vi "实时小时数据单参数上传.vi"() -> (4 "数据发送起始时间":timestamp format="%<%.3X\n%Y/%m/%d>T", 15 "error out":errorcluster)   [LabVIEW 2016, in "数据传输系统-04.lvlib"]
uses:
  <vilib>/Utility/config.llb/Read Key (String).vi
  <vilib>/Utility/config.llb/Write Key (String).vi
  <vilib>/Utility/config.llb/NI_LVConfig.lvlib
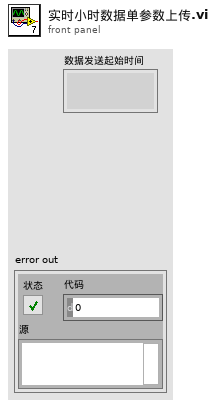
[diagram p1: front panel]
types:
  T1 = cluster{"CODMn":string, "CODCr":string, "DO":string, "铜":string, "PH":string, "氨氮":string, "比电导率":string, "水温":string, "COD":string, "浊度":string, "总氮":string, "总磷":string, "叶绿素a":string, "藻密度":string, "水位":string, "流速":string, "瞬时流量":string, "累积流量":string, "亚硝酸盐":string, "硫化物":string, "ORP":string, "铅":string, "镉":string, "锌":string, "镍":string, "锰":string, "汞":string, "气温":string, "气压":string, "风速":string, "风向":string, "盐度":string, "磷酸盐":string, "硝氮":string, "氟化物":string}
  T2 = cluster{"setini":string, "sysini":string, "hechaini":string, "actualwrite":string, "actualread":string, "datasent":string, "反控命令信息队列":string, "反控与仪器交互":string}
  T3 = typedef "NI_LVConfig.lvlib/Config Data RefNum.ctl" = refnum<k1>
  T4 = cluster{"time1":string, "time2":string, "time3":string, "time4":string, "time5":string, "time6":string, "time7":string, "time8":string, "time9":string, "time10":string, "time11":string, "time12":string, "time13":string, "time14":string, "time15":string, "time16":string, "time17":string, "time18":string, "time19":string, "time20":string, "time21":string, "time22":string, "time23":string, "time24":string, "time25":string, "time26":string, "time27":string, "time28":string, "time29":string, "time30":string, "time31":string, "time32":string, "time33":string, "time34":string, "time35":string}
  T5 = cluster{"水样数据索引[0]":string, "水样数据索引[1]":string, "水样数据索引[2]":string, "水样数据索引[3]":string, "水样数据索引[4]":string, "水样数据索引[5]":string, "水样数据索引[6]":string, "水样数据索引[7]":string, "水样数据索引[8]":string, "水样数据索引[9]":string, "水样数据索引[10]":string, "水样数据索引[11]":string, "水样数据索引[12]":string, "水样数据索引[13]":string, "水样数据索引[14]":string, "水样数据索引[15]":string, "水样数据索引[16]":string, "水样数据索引[17]":string, "水样数据索引[18]":string, "水样数据索引[19]":string, "水样数据索引[20]":string, "水样数据索引[21]":string, "水样数据索引[22]":string, "水样数据索引[23]":string, "水样数据索引[24]":string, "水样数据索引[25]":string, "水样数据索引[26]":string, "水样数据索引[27]":string, "水样数据索引[28]":string, "水样数据索引[29]":string, "水样数据索引[30]":string, "水样数据索引[31]":string, "水样数据索引[32]":string, "水样数据索引[33]":string, "水样数据索引[34]":string}
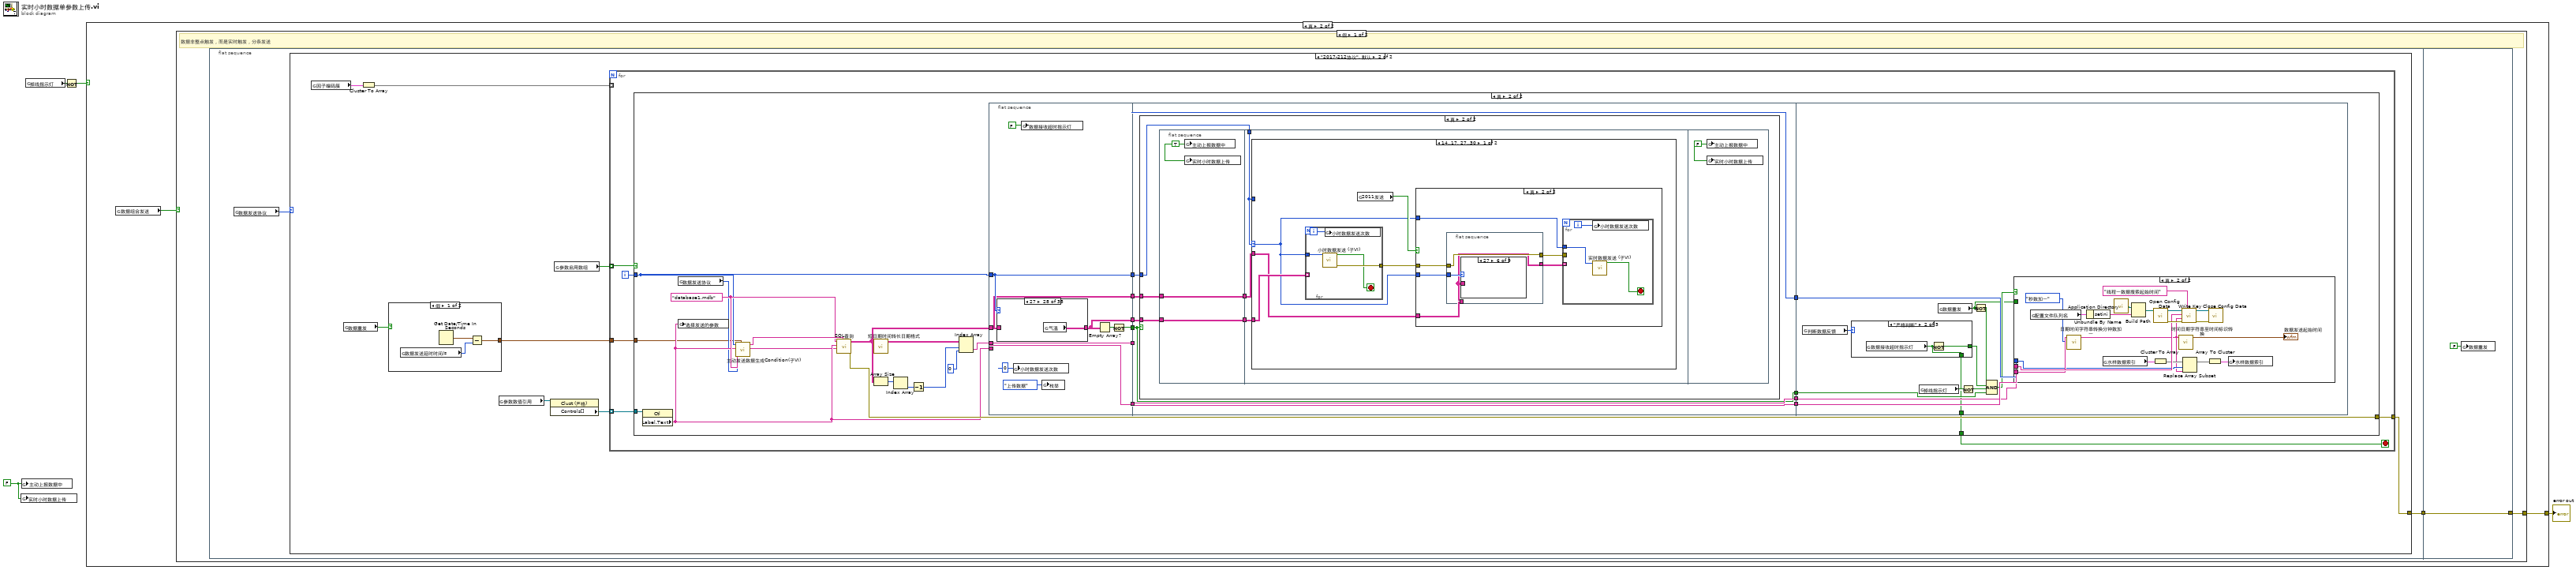
[diagram p0: block diagram]
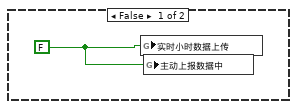
[diagram p2: hidden frame]
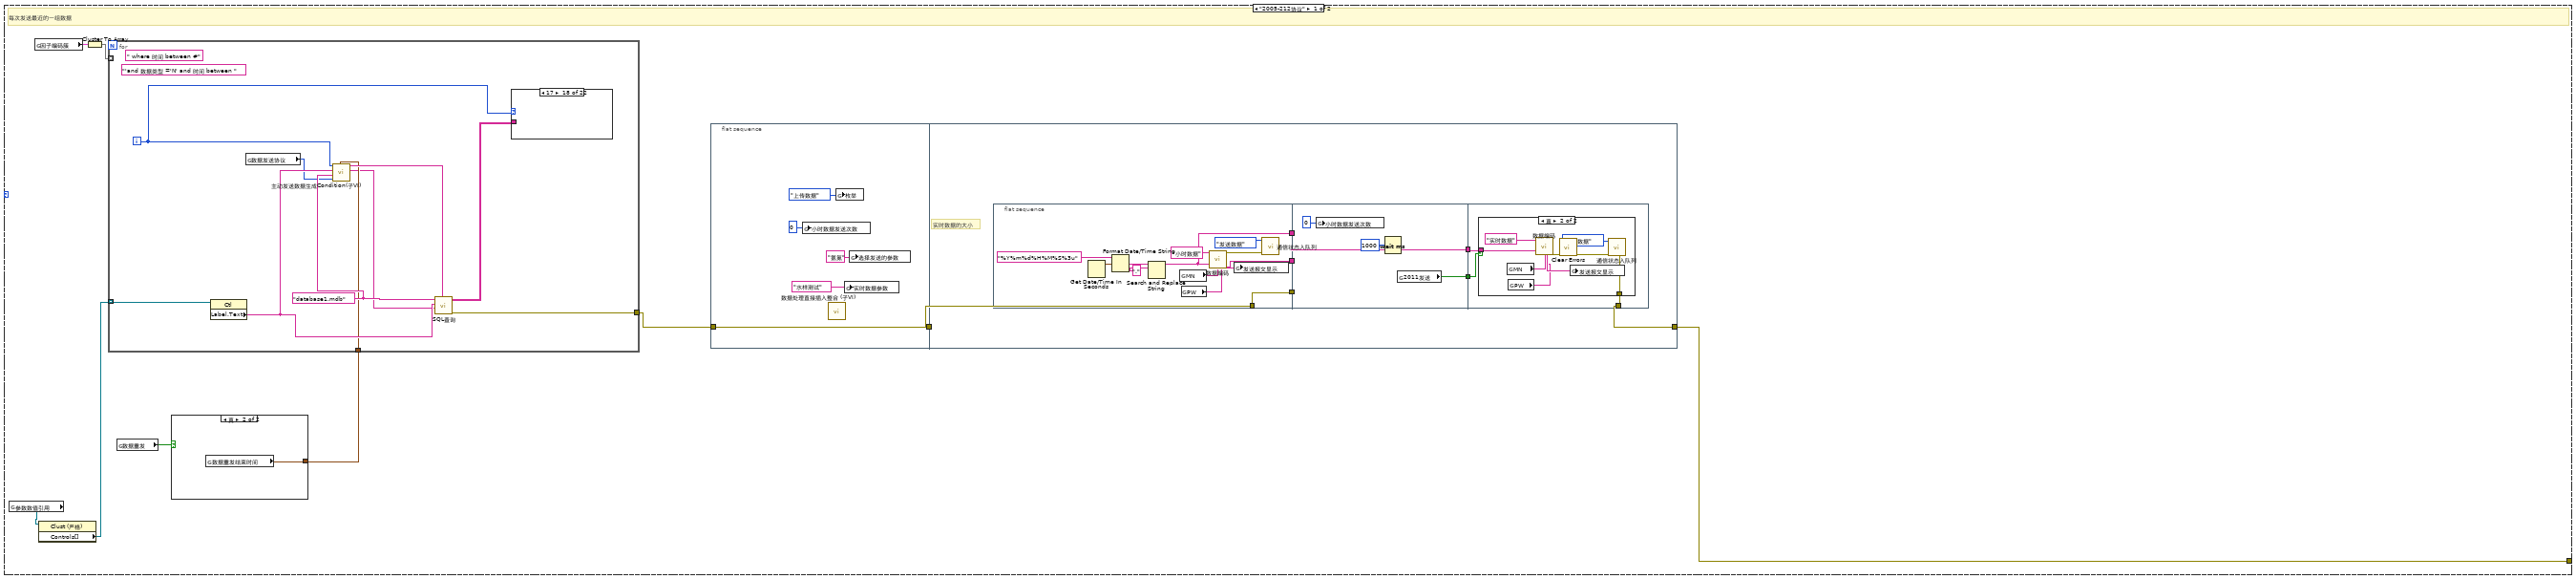
[diagram p3: hidden frame]
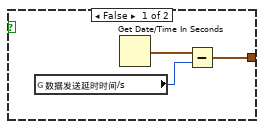
[diagram p4: hidden frame]
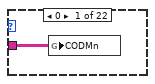
[diagram p6: hidden frame]
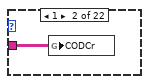
[diagram p7: hidden frame]
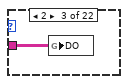
[diagram p8: hidden frame]
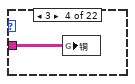
[diagram p9: hidden frame]
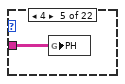
[diagram p10: hidden frame]
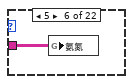
[diagram p11: hidden frame]
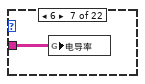
[diagram p12: hidden frame]
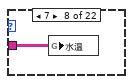
[diagram p13: hidden frame]
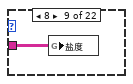
[diagram p14: hidden frame]
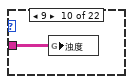
[diagram p15: hidden frame]
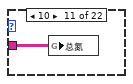
[diagram p16: hidden frame]
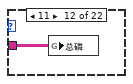
[diagram p17: hidden frame]
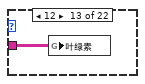
[diagram p18: hidden frame]
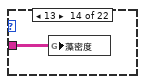
[diagram p19: hidden frame]
diagram:
  w1 = FALSE ("小时数据上传")
  n1 = global write "全局1.vi" "实时小时数据上传"(w1) -> ()
  n2 = global write "全局 数据发送重叠.vi" "主动上报数据中"(w1) -> ()
  n3 = global read "全局 数据发送重叠.vi" "掉线指示灯"() -> (w4:bool)
  n4 = Not(x=w4) -> (.not. x?=w3:bool)
  n5 = case shown="真" w3 {
    tunnel: [_ w7] -> w2
    frame False {
      w5 = FALSE ("小时数据上传")
      n6 = global write "全局1.vi" "实时小时数据上传"(w5) -> ()
      n7 = global write "全局 数据发送重叠.vi" "主动上报数据中"(w5) -> ()
    }
    frame True {
      n8 = global read "断电保存全局.vi" "数据组合发送"() -> (w6:bool)
      n9 = case shown="假" w6 {
        tunnel: [w8 _] -> w7
        frame False {
          # "数据非整点触发，而是实时触发，分条发送"
          n10 = flat-sequence {
            tunnel: [w11] -> w9
            tunnel: [w341] -> w8
            tunnel: w9 -> [w341]
            frame #0 {
              n11 = global read "断电保存全局.vi" "数据发送协议"() -> (w10:enum16{"2005-212协议", "2017-212协议"})
              n12 = case shown="\"2017-212协议\", 默认" w10 {
                tunnel: [w16 w98] -> w11
                frame "2005-212协议" {
                  # "每次发送最近的一组数据"
                  n13 = global read "断电保存全局.vi" "参数数值引用"() -> (w14:refnum<vi>)
                  n14 = global read "断电保存全局.vi" "因子编码簇"() -> (w15:T1)
                  n15 = property class="Clust (严格)"(reference=w14) -> ("Controls[]"=w17:refnum<vi>[])  [unwired: 1 in, 2 out]
                  n16 = Cluster To Array(cluster=w15) -> (array=w20:string[])
                  n17 = global read "断电保存全局.vi" "数据重发"() -> (w13:bool)
                  n18 = case shown="真" w13 {
                    tunnel: [w21 w24] -> w12
                    frame False {
                      n19 = global read "断电保存全局.vi" "数据发送延时时间/s"() -> (w22:i32)
                      n20 = Get Date/Time In Seconds() -> (seconds since 1Jan1904=w23:timestamp)
                      n21 = Subtract(x=w23, y=w22) -> (x-y=w21:timestamp)
                    }
                    frame True {
                      n22 = global read "断电保存全局.vi" "数据重发结束时间"() -> (w24:timestamp)
                    }
                  }
                  n23 = for {
                    tunnel: w20 -> [_] mode=indexing
                    tunnel: [w74] -> w19
                    tunnel: w17 -> [w69] mode=indexing
                    tunnel: w12 -> [w66]
                    i -> [w67]
                    (unwired) " where 时间 between #"
                    w72 = "database1.mdb" ("database")
                    (unwired) "'and 数据类型 ='N' and 时间 between "
                    n24 = property class="Ctl"(reference=w69) -> ("Label.Text"=w73:string)  [unwired: 1 in, 2 out]
                    n25 = global read "断电保存全局.vi" "数据发送协议"() -> (w70:enum16{"2005-212协议", "2017-212协议"})
                    n26 = call "主动发送数据生成Condition(子VI).vi"("结束时间"=w66, "数据发送协议"=w70, "database"=w72, "Label.Text"=w73, "数值"=w67) -> ("columns"=w65:string[], "CONDITION"=w71:string)  [unwired: 5 in]
                    n27 = call "SQL查询.vi"("condition"=w71, "columns"=w65, "table输入"=w73, "database"=w72) -> ("error out"=w74:errorcluster, "data"=w68:string[][])  [unwired: 5 in, 1 out]
                    n28 = case shown="17" w67 {
                      tunnel: w68 -> [w75 w76 w77 w78 w79 w80 w81 w82 w83 w84 w85 w86 w87 w88 _ _ _ _ w89 w90 w91 _]
                      frame 0 {
                        n29 = global write "全局 所有参数.vi" "CODMn"(w75) -> ()
                      }
                      frame 1 {
                        n30 = global write "全局 所有参数.vi" "CODCr"(w76) -> ()
                      }
                      frame 2 {
                        n31 = global write "全局 所有参数.vi" "DO"(w77) -> ()
                      }
                      frame 3 {
                        n32 = global write "全局 所有参数.vi" "铜"(w78) -> ()
                      }
                      frame 4 {
                        n33 = global write "全局 所有参数.vi" "PH"(w79) -> ()
                      }
                      frame 5 {
                        n34 = global write "全局 所有参数.vi" "氨氮"(w80) -> ()
                      }
                      frame 6 {
                        n35 = global write "全局 所有参数.vi" "电导率"(w81) -> ()
                      }
                      frame 7 {
                        n36 = global write "全局 所有参数.vi" "水温"(w82) -> ()
                      }
                      frame 8 {
                        n37 = global write "全局 所有参数.vi" "盐度"(w83) -> ()
                      }
                      frame 9 {
                        n38 = global write "全局 所有参数.vi" "浊度"(w84) -> ()
                      }
                      frame 10 {
                        n39 = global write "全局 所有参数.vi" "总氮"(w85) -> ()
                      }
                      frame 11 {
                        n40 = global write "全局 所有参数.vi" "总磷"(w86) -> ()
                      }
                      frame 12 {
                        n41 = global write "全局 所有参数.vi" "叶绿素"(w87) -> ()
                      }
                      frame 13 {
                        n42 = global write "全局 所有参数.vi" "藻密度"(w88) -> ()
                      }
                      frame 14 {
                      }
                      frame 15 {
                      }
                      frame 16 {
                      }
                      frame 17 {
                      }
                      frame 18 {
                        n43 = global write "全局 所有参数.vi" "亚硝酸盐"(w89) -> ()
                      }
                      frame 19 {
                        n44 = global write "全局 所有参数.vi" "硫化物"(w90) -> ()
                      }
                      frame 20 {
                        n45 = global write "全局 所有参数.vi" "ORP"(w91) -> ()
                      }
                      frame 21, Default {
                      }
                    }
                  }
                  n46 = flat-sequence {
                    tunnel: w19 -> [w25]
                    tunnel: [w25] -> w18
                    tunnel: w18 -> [w34]
                    tunnel: [w33] -> w16
                    frame #0 {
                      n47 = global write "全局 小时数据发送次数.vi" "小时数据发送次数"(0 ("小时数据发送次数")) -> ()
                      n48 = call "数据处理直接插入整合 (子VI).vi"() -> ()  [unwired: 12 in]
                      n49 = global write "全局1.vi" "枚举"(enum16{"返回请求应答", "上传数据", "返回执行结果"}."上传数据" ("枚举")) -> ()
                      n50 = global write "全局 实时数据参数.vi" "实时数据参数"("水样测试" ("实时数据参数")) -> ()
                      n51 = global write "全局 水样时间.vi" "选择发送的参数"("氨氮" ("选择发送的参数")) -> ()
                    }
                    frame #1 {
                      # "实时数据的大小"
                      n52 = flat-sequence {
                        tunnel: [w43] -> w36
                        tunnel: [w38] -> w35
                        tunnel: w34 -> [w38]
                        tunnel: [w37] -> w32
                        tunnel: w36 -> [_]
                        tunnel: w35 -> [_]
                        tunnel: w32 -> [w50]
                        tunnel: [w50] -> w31
                        tunnel: [w49] -> w30
                        tunnel: [w55] -> w33
                        tunnel: w31 -> [w54]
                        tunnel: w30 -> [w53]
                        frame #0 {
                          n53 = Get Date/Time In Seconds() -> (seconds since 1Jan1904=w46:timestamp)
                          n54 = Format Date/Time String(time format string (%c)="%Y%m%d%H%M%S%3u" ("时间格式字符串(%c)"), seconds (now)=w46) -> (date/time string=w47:string)  [unwired: 1 in]
                          n55 = Search and Replace String(input string=w47, search string="." ("搜索字符串")) -> (result string=w37:string)  [unwired: 6 in, 3 out]
                          n56 = global read "断电保存全局.vi" "MN"() -> (w41:string)
                          n57 = global read "断电保存全局.vi" "PW"() -> (w40:string)
                          n58 = call "数据编码.vi"("table输入"="小时数据" ("新元素/子数组"), "QN"=w37, "MN"=w41, "PW"=w40) -> ("错误常量"=w39:errorcluster, "通讯包字符串"=w43:string)  [unwired: 10 in]
                          n59 = global write "全局1.vi" "发送报文显示"(w43) -> ()
                          n60 = call "通信状态入队列.vi"("错误输入（无错误）"=w39, "枚举"=enum16{"打开连接", "发送数据", "读取数据", "数据处理", "关闭连接"}."发送数据") -> ()  [unwired: 9 in, 1 out]
                        }
                        frame #1 {
                          n61 = global write "全局 小时数据发送次数.vi" "小时数据发送次数"(0 ("小时数据发送次数")) -> ()
                          n62 = Wait (ms)(milliseconds to wait=u32 1000 ("等待时间（毫秒）")) -> ()  [unwired: 1 out]
                          n63 = global read "断电保存全局.vi" "2011发送"() -> (w49:bool)
                        }
                        frame #2 {
                          n64 = case shown="真" w53 {
                            tunnel: [_ w58] -> w55
                            tunnel: w54 -> [_ w57]
                            frame False {
                            }
                            frame True {
                              n65 = global read "断电保存全局.vi" "MN"() -> (w60:string)
                              n66 = global read "断电保存全局.vi" "PW"() -> (w61:string)
                              n67 = call "数据编码.vi"("table输入"="实时数据" ("新元素/子数组"), "QN"=w57, "MN"=w60, "PW"=w61) -> ("错误常量"=w59:errorcluster, "通讯包字符串"=w63:string)  [unwired: 10 in]
                              n68 = call <vilib>:"Clear Errors.vi"("error in (no error)"=w59) -> ("error out"=w56:errorcluster)  [unwired: 5 in, 1 out]
                              n69 = global write "全局1.vi" "发送报文显示"(w63) -> ()
                              n70 = call "通信状态入队列.vi"("错误输入（无错误）"=w56, "枚举"=enum16{"打开连接", "发送数据", "读取数据", "数据处理", "关闭连接"}."发送数据") -> ("错误输出"=w58:errorcluster)  [unwired: 9 in]
                            }
                          }
                        }
                      }
                    }
                  }
                }
                frame "2017-212协议", Default {
                  n71 = global read "断电保存全局.vi" "因子编码簇"() -> (w96:T1)
                  n72 = global read "断电保存全局.vi" "数据重发"() -> (w93:bool)
                  n73 = Cluster To Array(cluster=w96) -> (array=w99:string[])
                  n74 = case shown="假" w93 {
                    tunnel: [w100 w103] -> w92
                    frame False {
                      n75 = global read "断电保存全局.vi" "数据发送延时时间/s"() -> (w101:i32)
                      n76 = Get Date/Time In Seconds() -> (seconds since 1Jan1904=w102:timestamp)
                      n77 = Subtract(x=w102, y=w101) -> (x-y=w100:timestamp)
                    }
                    frame True {
                      n78 = global read "断电保存全局.vi" "数据重发结束时间"() -> (w103:timestamp)
                    }
                  }
                  n79 = global read "断电保存全局.vi" "参数数值引用"() -> (w95:refnum<vi>)
                  n80 = property class="Clust (严格)"(reference=w95) -> ("Controls[]"=w97:refnum<vi>[])  [unwired: 1 in, 2 out]
                  n81 = global read "断电保存全局.vi" "参数启用数组"() -> (w94:bool[])
                  n82 = for {
                    tunnel: w99 -> [_] mode=indexing
                    tunnel: [w109] -> w98
                    tunnel: w97 -> [w107] mode=indexing
                    tunnel: w94 -> [w106] mode=indexing
                    tunnel: w92 -> [w105]
                    i -> [w108]
                    stop <- w104 stop-if-true
                    n83 = case shown="真" w106 {
                      tunnel: [_ w125] -> w109
                      tunnel: w108 -> [_ w116]
                      tunnel: w107 -> [_ w115]
                      tunnel: w105 -> [_ w112]
                      tunnel: [_ w110] -> w104
                      frame False {
                      }
                      frame True {
                        w124 = "database1.mdb" ("database")
                        n84 = property class="Ctl"(reference=w115) -> ("Label.Text"=w123:string)  [unwired: 1 in, 2 out]
                        n85 = global read "断电保存全局.vi" "数据发送协议"() -> (w122:enum16{"2005-212协议", "2017-212协议"})
                        n86 = global write "全局 水样时间.vi" "选择发送的参数"(w123) -> ()
                        n87 = call "主动发送数据生成Condition(子VI).vi"("结束时间"=w112, "数据发送协议"=w122, "database"=w124, "Label.Text"=w123, "数值"=w116) -> ("columns"=w114:string[], "CONDITION"=w128:string)  [unwired: 5 in]
                        n88 = call "SQL查询.vi"("condition"=w128, "columns"=w114, "table输入"=w123, "database"=w124) -> ("error out"=w125:errorcluster, "data"=w119:string[][])  [unwired: 5 in, 1 out]
                        n89 = call "短日期时间转长日期格式.vi"("data"=w119) -> ("输出数组"=w127:string[][])  [unwired: 10 in]
                        n90 = Array Size(array=w119) -> (size(s)=w121:i32[])
                        n91 = Index Array(array=w121) -> (element=w120:i32)  [unwired: 1 in]
                        n92 = Decrement(x=w120) -> (x-1=w118:i32)
                        n93 = Index Array(array=w127, index (row)=w118, index (col)=0 ("禁用的索引 (列)")) -> (element=w126:string)
                        n94 = flat-sequence {
                          tunnel: [w139] -> w136
                          tunnel: [w138] -> w135
                          tunnel: w119 -> [w137]
                          tunnel: w116 -> [w142]
                          tunnel: w123 -> [w144]
                          tunnel: [w144] -> w134
                          tunnel: w126 -> [w143]
                          tunnel: [w143] -> w133
                          tunnel: [w142] -> w132
                          tunnel: [w137] -> w111
                          tunnel: w136 -> [w183]
                          tunnel: w135 -> [w187]
                          tunnel: [w186] -> w131
                          tunnel: w134 -> [w186]
                          tunnel: [w185] -> w130
                          tunnel: w133 -> [w185]
                          tunnel: [w184] -> w129
                          tunnel: w132 -> [w184]
                          tunnel: [w183] -> w113
                          tunnel: w111 -> [w182]
                          tunnel: w131 -> [w295]
                          tunnel: w130 -> [w294]
                          tunnel: w129 -> [w293]
                          tunnel: w113 -> [w292]
                          tunnel: [w284] -> w110
                          frame #0 {
                            n95 = case shown="27" w142 {
                              tunnel: w137 -> [w147 w148 w149 w150 w151 w152 w153 w154 w155 w156 w157 w158 w159 w160 _ _ _ _ w165 w166 w167 w168 w169 w170 w171 w172 w173 _ _ _ _ w178 w179 w180 w181]
                              tunnel: [w147 w148 w149 w150 w151 w152 w153 w154 w155 w156 w157 w158 w159 w160 w161 w162 w163 w164 w165 w166 w167 w168 w169 w170 w171 w172 w173 w174 w175 w176 w177 w178 w179 w180 w181] -> w138
                              frame 0, Default {
                                n96 = global write "全局 所有参数.vi" "CODMn"(w147) -> ()
                              }
                              frame 1 {
                                n97 = global write "全局 所有参数.vi" "CODCr"(w148) -> ()
                              }
                              frame 2 {
                                n98 = global write "全局 所有参数.vi" "DO"(w149) -> ()
                              }
                              frame 3 {
                                n99 = global write "全局 所有参数.vi" "铜"(w150) -> ()
                              }
                              frame 4 {
                                n100 = global write "全局 所有参数.vi" "PH"(w151) -> ()
                              }
                              frame 5 {
                                n101 = global write "全局 所有参数.vi" "氨氮"(w152) -> ()
                              }
                              frame 6 {
                                n102 = global write "全局 所有参数.vi" "电导率"(w153) -> ()
                              }
                              frame 7 {
                                n103 = global write "全局 所有参数.vi" "水温"(w154) -> ()
                              }
                              frame 8 {
                                n104 = global write "全局 所有参数.vi" "盐度"(w155) -> ()
                              }
                              frame 9 {
                                n105 = global write "全局 所有参数.vi" "浊度"(w156) -> ()
                              }
                              frame 10 {
                                n106 = global write "全局 所有参数.vi" "总氮"(w157) -> ()
                              }
                              frame 11 {
                                n107 = global write "全局 所有参数.vi" "总磷"(w158) -> ()
                              }
                              frame 12 {
                                n108 = global write "全局 所有参数.vi" "叶绿素"(w159) -> ()
                              }
                              frame 13 {
                                n109 = global write "全局 所有参数.vi" "藻密度"(w160) -> ()
                              }
                              frame 14 {
                                n110 = global read "全局 所有参数.vi" "水位"() -> (w161:string[][])
                              }
                              frame 15 {
                                n111 = global read "全局 所有参数.vi" "流速"() -> (w162:string[][])
                              }
                              frame 16 {
                                n112 = global read "全局 所有参数.vi" "瞬时流量"() -> (w163:string[][])
                              }
                              frame 17 {
                                n113 = global read "全局 所有参数.vi" "累积流量"() -> (w164:string[][])
                              }
                              frame 18 {
                                n114 = global write "全局 所有参数.vi" "亚硝酸盐"(w165) -> ()
                              }
                              frame 19 {
                                n115 = global write "全局 所有参数.vi" "硫化物"(w166) -> ()
                              }
                              frame 20 {
                                n116 = global write "全局 所有参数.vi" "ORP"(w167) -> ()
                              }
                              frame 21 {
                                n117 = global write "全局 所有参数.vi" "铅"(w168) -> ()
                              }
                              frame 22 {
                                n118 = global write "全局 所有参数.vi" "镉"(w169) -> ()
                              }
                              frame 23 {
                                n119 = global write "全局 所有参数.vi" "锌"(w170) -> ()
                              }
                              frame 24 {
                                n120 = global write "全局 所有参数.vi" "镍"(w171) -> ()
                              }
                              frame 25 {
                                n121 = global write "全局 所有参数.vi" "锰"(w172) -> ()
                              }
                              frame 26 {
                                n122 = global write "全局 所有参数.vi" "汞"(w173) -> ()
                              }
                              frame 27 {
                                n123 = global read "全局 所有参数.vi" "气温"() -> (w174:string[][])
                              }
                              frame 28 {
                                n124 = global read "全局 所有参数.vi" "气压"() -> (w175:string[][])
                              }
                              frame 29 {
                                n125 = global read "全局 所有参数.vi" "风速"() -> (w176:string[][])
                              }
                              frame 30 {
                                n126 = global read "全局 所有参数.vi" "风向"() -> (w177:string[][])
                              }
                              frame 31 {
                                n127 = global write "全局 所有参数.vi" "盐度 2"(w178) -> ()
                              }
                              frame 32 {
                                n128 = global write "全局 所有参数.vi" "磷酸盐"(w179) -> ()
                              }
                              frame 33 {
                                n129 = global write "全局 所有参数.vi" "硝氮"(w180) -> ()
                              }
                              frame 34 {
                                n130 = global write "全局 所有参数.vi" "氟化物"(w181) -> ()
                              }
                            }
                            n131 = global write "全局 小时数据发送次数.vi" "小时数据发送次数"(0 ("小时数据发送次数")) -> ()
                            n132 = global write "全局 数据发送重叠.vi" "数据接收超时指示灯"(FALSE ("数据接收超时指示灯")) -> ()
                            n133 = global write "全局1.vi" "枚举"(enum16{"返回请求应答", "上传数据", "返回执行结果"}."上传数据" ("枚举")) -> ()
                            n134 = Empty Array?(array=w138) -> (empty?=w140:bool)
                            n135 = Not(x=w140) -> (.not. x?=w139:bool)
                          }
                          frame #1 {
                            n136 = case shown="真" w183 {
                              tunnel: w187 -> [_ w192]
                              tunnel: w184 -> [_ w191]
                              tunnel: w182 -> [_ w189]
                              frame False {
                              }
                              frame True {
                                n137 = flat-sequence {
                                tunnel: w192 -> [w195]
                                tunnel: [w195] -> w190
                                tunnel: w189 -> [w193]
                                tunnel: [w193] -> w188
                                tunnel: w191 -> [w197]
                                tunnel: w190 -> [w198]
                                tunnel: w188 -> [w196]
                                frame #0 {
                                w194 = TRUE ("小时数据上传")
                                n138 = global write "全局 数据发送重叠.vi" "主动上报数据中"(w194) -> ()
                                n139 = global write "全局1.vi" "实时小时数据上传"(w194) -> ()
                                }
                                frame #1 {
                                n140 = case shown="14..17, 27..30" w197 {
                                selector: w197 -> [w199 _]
                                tunnel: w197 -> [_ w230]
                                tunnel: w198 -> [w202 w229]
                                tunnel: w196 -> [w201 w228]
                                frame 14..17, 27..30 {
                                n141 = for {
                                tunnel: [w226] -> w203
                                tunnel: w199 -> [w225]
                                tunnel: w202 -> [_] mode=indexing
                                i -> [w227]
                                stop <- w224 stop-if-true
                                n142 = call "小时数据发送 (子VI).vi"("数值"=w225) -> ("error out"=w226:errorcluster, "超时退出"=w224:bool)  [unwired: 9 in]
                                n143 = global write "全局 小时数据发送次数.vi" "小时数据发送次数"(w227) -> ()
                                }
                                n144 = global read "断电保存全局.vi" "2011发送"() -> (w200:bool)
                                n145 = case shown="真" w200 {
                                tunnel: w203 -> [_ w208]
                                tunnel: w199 -> [_ w207]
                                tunnel: w201 -> [_ w206]
                                tunnel: w199 -> [_ w204]
                                frame False {
                                }
                                frame True {
                                n146 = flat-sequence {
                                tunnel: w208 -> [w212]
                                tunnel: [w212] -> w209
                                tunnel: w207 -> [w211]
                                tunnel: w206 -> [w210]
                                tunnel: [w210] -> w205
                                frame #0 {
                                n147 = case shown="27" w211 {
                                tunnel: w210 -> [_ w213 w214 w215 w216 w217 w218 w219 w220]
                                frame 0, Default {
                                }
                                frame 14 {
                                n148 = global write "全局 所有参数.vi" "水位"(w213) -> ()
                                }
                                frame 15 {
                                n149 = global write "全局 所有参数.vi" "流速"(w214) -> ()
                                }
                                frame 16 {
                                n150 = global write "全局 所有参数.vi" "瞬时流量"(w215) -> ()
                                }
                                frame 17 {
                                n151 = global write "全局 所有参数.vi" "累积流量"(w216) -> ()
                                }
                                frame 27 {
                                n152 = global write "全局 所有参数.vi" "气温"(w217) -> ()
                                }
                                frame 28 {
                                n153 = global write "全局 所有参数.vi" "气压"(w218) -> ()
                                }
                                frame 29 {
                                n154 = global write "全局 所有参数.vi" "风速"(w219) -> ()
                                }
                                frame 30 {
                                n155 = global write "全局 所有参数.vi" "风向"(w220) -> ()
                                }
                                }
                                }
                                }
                                n156 = for {
                                tunnel: w209 -> [_]
                                tunnel: w205 -> [_] mode=indexing
                                tunnel: w204 -> [w222]
                                i -> [w223]
                                stop <- w221 stop-if-true
                                n157 = global write "全局 小时数据发送次数.vi" "小时数据发送次数"(w223) -> ()
                                n158 = call "实时数据发送 (子VI).vi"("数值"=w222) -> ("超时退出"=w221:bool)  [unwired: 10 in]
                                }
                                }
                                }
                                }
                                frame 0, Default {
                                n159 = for {
                                tunnel: w230 -> [w233]
                                tunnel: w229 -> [w239] mode=indexing
                                tunnel: w228 -> [w235]
                                i -> [w234]
                                stop <- w231 stop-if-true
                                n160 = Index Array(array=w239, index #1=1 ("索引"), index #2=2 ("索引")) -> (element #1=w232:string, element #2=w236:string)
                                n161 = global write "全局 小时数据发送次数.vi" "小时数据发送次数"(w234) -> ()
                                n162 = case shown="\"水样测试\"" w232 {
                                tunnel: w233 -> [_ w243 _ _ _]
                                tunnel: w236 -> [_ w242 w275 w278 w281]
                                tunnel: w235 -> [_ w241 _ _ _]
                                tunnel: [_ w240 w274 w277 w280] -> w231
                                frame "假", Default {
                                }
                                frame "水样测试" {
                                n163 = case shown="\"hd\", \"N\", 默认" w242 {
                                tunnel: w243 -> [w247 w268]
                                tunnel: w241 -> [w246 w267]
                                tunnel: [w244 w265] -> w240
                                frame "M" {
                                n164 = global read "断电保存全局.vi" "2011发送"() -> (w245:bool)
                                n165 = case shown="真" w245 {
                                tunnel: w247 -> [_ w250]
                                tunnel: w246 -> [_ w249]
                                tunnel: [_ w248] -> w244
                                frame False {
                                }
                                frame True {
                                n166 = flat-sequence {
                                tunnel: w250 -> [w252]
                                tunnel: w249 -> [w253]
                                tunnel: [w252] -> w251
                                tunnel: w251 -> [w263]
                                tunnel: [w262] -> w248
                                frame #0 {
                                n167 = case shown="14" w252 {
                                tunnel: w253 -> [_ w254 w255 w256 w257 w258 w259 w260 w261]
                                frame 0, Default {
                                }
                                frame 14 {
                                n168 = global write "全局 所有参数.vi" "水位"(w254) -> ()
                                }
                                frame 15 {
                                n169 = global write "全局 所有参数.vi" "流速"(w255) -> ()
                                }
                                frame 16 {
                                n170 = global write "全局 所有参数.vi" "瞬时流量"(w256) -> ()
                                }
                                frame 17 {
                                n171 = global write "全局 所有参数.vi" "累积流量"(w257) -> ()
                                }
                                frame 27 {
                                n172 = global write "全局 所有参数.vi" "气温"(w258) -> ()
                                }
                                frame 28 {
                                n173 = global write "全局 所有参数.vi" "气压"(w259) -> ()
                                }
                                frame 29 {
                                n174 = global write "全局 所有参数.vi" "风速"(w260) -> ()
                                }
                                frame 30 {
                                n175 = global write "全局 所有参数.vi" "风向"(w261) -> ()
                                }
                                }
                                }
                                frame #1 {
                                n176 = call "实时数据发送 (子VI).vi"("数值"=w263) -> ("超时退出"=w262:bool)  [unwired: 10 in]
                                }
                                }
                                }
                                }
                                }
                                frame "hd", "N", Default {
                                n177 = call "小时数据发送 (子VI).vi"("数值"=w268) -> ("error out"=w266:errorcluster, "超时退出"=w264:bool)  [unwired: 9 in]
                                n178 = global read "断电保存全局.vi" "2011发送"() -> (w269:bool)
                                n179 = case shown="真" w269 {
                                tunnel: w268 -> [_ w273]
                                tunnel: w267 -> [_ _]
                                tunnel: w266 -> [_ _]
                                tunnel: [_ w270] -> w265
                                tunnel: w264 -> [_ w272]
                                frame False {
                                }
                                frame True {
                                n180 = call "实时数据发送 (子VI).vi"("数值"=w273) -> ("超时退出"=w271:bool)  [unwired: 10 in]
                                n181 = Or(x=w272, y=w271) -> (x .or. y?=w270:bool)
                                }
                                }
                                }
                                }
                                }
                                frame "空白测试", "零点核查" {
                                n182 = case shown="\"N\", 默认" w275 {
                                tunnel: [_ w276] -> w274
                                frame "M" {
                                }
                                frame "N", Default {
                                n183 = call "零点核查数据发送 (子VI).vi"() -> ("超时退出"=w276:bool)  [unwired: 11 in]
                                }
                                }
                                }
                                frame "跨度核查" {
                                n184 = case shown="\"N\", 默认" w278 {
                                tunnel: [_ w279] -> w277
                                frame "M" {
                                }
                                frame "N", Default {
                                n185 = call "跨度核查数据发送 (子VI).vi"() -> ("超时退出"=w279:bool)  [unwired: 11 in]
                                }
                                }
                                }
                                frame "标样核查" {
                                n186 = case shown="\"N\", 默认" w281 {
                                tunnel: [_ w282] -> w280
                                frame "M" {
                                }
                                frame "N", Default {
                                n187 = call "标样核查数据发送(子VI).vi"() -> ("超时退出"=w282:bool)  [unwired: 11 in]
                                }
                                }
                                }
                                }
                                }
                                }
                                }
                                }
                                frame #2 {
                                w283 = FALSE ("小时数据上传")
                                n188 = global write "全局 数据发送重叠.vi" "主动上报数据中"(w283) -> ()
                                n189 = global write "全局1.vi" "实时小时数据上传"(w283) -> ()
                                }
                                }
                              }
                            }
                          }
                          frame #2 {
                            n190 = global read "断电保存全局.vi" "判断数据反馈"() -> (w289:enum16{"非严格判断", "严格判断", "不判断"})
                            n191 = case shown="\"严格判断\"" w289 {
                              tunnel: [TRUE w299 TRUE] -> w288
                              tunnel: [FALSE ("数据接收超时指示灯") w298 FALSE ("数据接收超时指示灯")] -> w284
                              frame "非严格判断", Default {
                              }
                              frame "严格判断" {
                                n192 = global read "全局 数据发送重叠.vi" "数据接收超时指示灯"() -> (w298:bool)
                                n193 = Not(x=w298) -> (.not. x?=w299:bool)
                              }
                              frame "不判断" {
                              }
                            }
                            n194 = global read "全局 数据发送重叠.vi" "掉线指示灯"() -> (w291:bool)
                            n195 = global read "断电保存全局.vi" "数据重发"() -> (w285:bool)
                            n196 = Not(x=w291) -> (.not. x?=w290:bool)
                            n197 = Not(x=w285) -> (.not. x?=w286:bool)
                            n198 = Compound Arithmetic op=AND ("复合运算")(w286, w288, w290, w292) -> (w287:bool)
                            n199 = case shown="真" w287 {
                              tunnel: w294 -> [_ w331]
                              tunnel: w293 -> [w302 w325]
                              tunnel: w295 -> [w304 w332]
                              tunnel: w285 -> [w303 _]
                              frame False {
                                n200 = case shown="假" w303 {
                                tunnel: w304 -> [_ w307]
                                tunnel: w302 -> [_ w305]
                                frame False {
                                }
                                frame True {
                                n201 = global read "断电保存全局.vi" "配置文件队列名"() -> (w314:T2)
                                n202 = Unbundle By Name(w314) -> ("setini"=w315:string)
                                n203 = call <vilib>:"Application Directory.vi"() -> ("Application Directory"=w308:path)
                                n204 = Build Path(base path=w308, name or relative path=w315) -> (appended path=w309:path)
                                n205 = call <vilib>:"Open Config Data.vi"("configuration file path"=w309) -> ("error out"=w316:errorcluster, "refnum"=w310:T3)  [unwired: 8 in, 1 out]
                                n206 = global read "全局 水样时间.vi" "水样数据索引"() -> (w317:T4)
                                n207 = call-poly <vilib>:"Read Key.vi"("section"="线程一数据搜索起始时间", "error in (no error)"=w316, "key"=w307, "refnum"=w310) -> ("error out"=w313:errorcluster, "value"=w306:string, "refnum out"=w312:T3)  [unwired: 4 in, 1 out]
                                n208 = Cluster To Array(cluster=w317) -> (array=w318:string[])
                                n209 = call <vilib>:"Close Config Data.vi"("error in (no error)"=w313, "refnum"=w312) -> ()  [unwired: 8 in, 2 out]
                                n210 = Replace Array Subset(array=w318, new element=w306, index=w305) -> (w319:string[])
                                n211 = Array To Cluster(array=w319) -> (cluster=w320:T5)
                                n212 = global write "全局 水样时间.vi" "水样数据索引"(w320) -> ()
                                }
                                }
                              }
                              frame True {
                                n213 = global read "断电保存全局.vi" "配置文件队列名"() -> (w322:T2)
                                n214 = call "日期时间字符串转换分钟数加一.vi"("枚举"=enum16{"分钟数加一", "秒数加一", "小时数加一"}."秒数加一", "data[0]"=w331) -> ("日期/时间字符串"=w324:string)  [unwired: 9 in]
                                n215 = Unbundle By Name(w322) -> ("setini"=w321:string)
                                n216 = global read "全局 水样时间.vi" "水样数据索引"() -> (w326:T4)
                                n217 = call <vilib>:"Application Directory.vi"() -> ("Application Directory"=w333:path)
                                n218 = Build Path(base path=w333, name or relative path=w321) -> (appended path=w334:path)
                                n219 = Cluster To Array(cluster=w326) -> (array=w327:string[])
                                n220 = call <vilib>:"Open Config Data.vi"("configuration file path"=w334) -> ("error out"=w336:errorcluster, "refnum"=w335:T3)  [unwired: 8 in, 1 out]
                                n221 = call "时间日期字符串至时间标识转换.vi"("时间日期字符串"=w324) -> ("时间标识"=→"数据发送起始时间":timestamp)  [unwired: 10 in]
                                n222 = call-poly <vilib>:"Write Key.vi"("section"="线程一数据搜索起始时间", "error in (no error)"=w336, "value"=w324, "key"=w332, "refnum"=w335) -> ("error out"=w338:errorcluster, "refnum out"=w337:T3)  [unwired: 4 in, 1 out]
                                n223 = Replace Array Subset(array=w327, new element=w324, index=w325) -> (w328:string[])
                                n224 = Array To Cluster(array=w328) -> (cluster=w329:T5)
                                n225 = call <vilib>:"Close Config Data.vi"("error in (no error)"=w338, "refnum"=w337) -> ()  [unwired: 8 in, 2 out]
                                n226 = global write "全局 水样时间.vi" "水样数据索引"(w329) -> ()
                              }
                            }
                          }
                        }
                      }
                    }
                  }
                }
              }
            }
            frame #1 {
              n227 = global write "断电保存全局.vi" "数据重发"(FALSE ("数据重发")) -> ()
            }
          }
        }
        frame True {
          # "数据整点触发，整条发送"
          n228 = flat-sequence {
            frame #0 {
              n229 = global read "断电保存全局.vi" "数据发送通道"() -> (w342:enum16{"TCP", "VISA"})
              n230 = global read "断电保存全局.vi" "MN"() -> (w344:string)
              n231 = global read "断电保存全局.vi" "PW"() -> (w343:string)
              n232 = call "数据全参数一起发送整点触发.vi"("数据发送通道"=w342, "PW"=w343, "MN"=w344) -> ()  [unwired: 8 in]
            }
            frame #1 {
              w345 = FALSE ("主动上报数据中")
              n233 = global write "全局 数据发送重叠.vi" "主动上报数据中"(w345) -> ()
              n234 = global write "全局1.vi" "实时小时数据上传"(w345) -> ()
            }
          }
        }
      }
    }
  }
  "error out" <- w2
